vi "Start.vi"(8 "error in (no error)":errorcluster, 10 "Message in":refnum<class "StartMessage.lvclass">, 11 "Waveform in":refnum<class "Waveform.lvclass">) -> (0 "error out":errorcluster, 3 "Waveform out":refnum<class "Waveform.lvclass">)   [LabVIEW 2012, in "Waveform.lvclass"]
doc: "This member function is called when the statemachine in the run.vi receives an 'start' command. It relays the message to all observers of the component.\n\nOverride this member function in your derived class if you need additional start functionality (but don't forget to call the parent method)."
uses:
  Waveform.lvclass
  <vilib>/Distrio/Murmex/StartMessage/StartMessage.lvclass
  <vilib>/Distrio/Murmex/Murmex/Murmex.lvclass
  <vilib>/Distrio/Murmex/StartMessage/run mode enum.ctl
  Waveform.lvclass/Waveform.ctl
  <vilib>/Distrio/Murmex/StartMessage/Get run mode.vi
  <vilib>/Distrio/Murmex/Message/Message.lvclass
panel:
  # "This member function is called when the statemachine in the run.vi receives an 'start' command. It relays the message to all observers of the component.\n\nOverride this member function in your derived class if you need additional start functionality (but don't forget to call the parent method)."
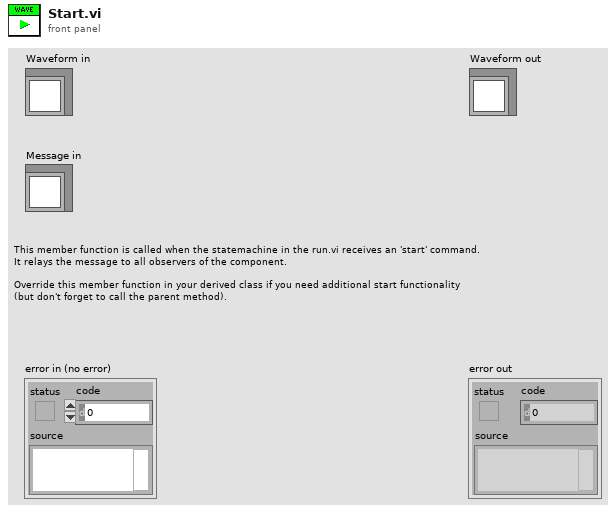
[diagram p1: front panel]
types:
  T1 = enum8{"Enabled", "Disabled", "Disabled and Grayed Out"}
  T2 = typedef "Murmex.lvlib/StartMessage.lvclass/run mode enum.ctl" = enum16{"infinite", "finite"}
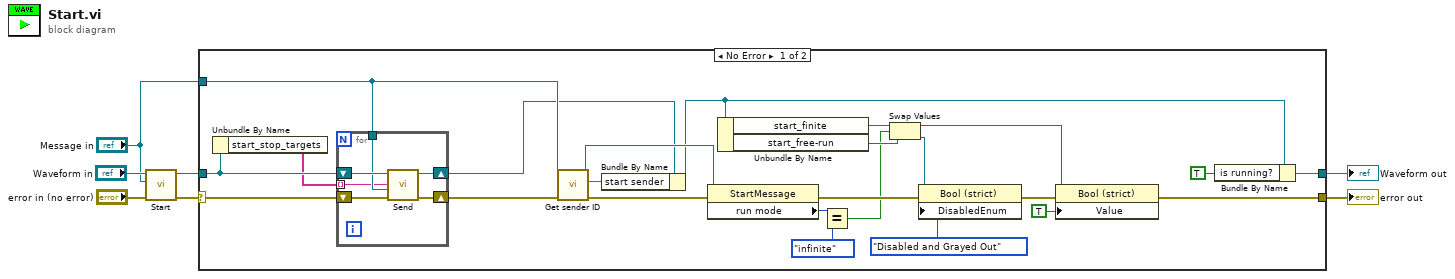
[diagram p0: block diagram]
diagram:
  n1 = call-parent "Start.vi"("error in (no error)"="error in (no error)", "Message in"="Message in", "Murmex in"="Waveform in") -> ("error out"=w5:errorcluster, "Murmex out"=w4:refnum<class "Waveform.lvclass">)  [unwired: 7 in]
  n2 = case shown="No Error" w5 {
    selector: w5 -> [w16 w39]
    tunnel: w4 -> [w14 w38]
    tunnel: [w9 w39] -> w3
    tunnel: [w17 w38] -> w2
    tunnel: "Message in" -> [w15 _]
    frame No Error {
      n3 = Unbundle By Name(w14) -> ("start_stop_targets"=w13:string[])
      n4 = for {
        shift-right: [w36] -> w11
        shift-left: w16 -> [w37]
        shift-right: [w34] -> w10
        shift-left: w14 -> [w35]
        tunnel: w15 -> [w33]
        tunnel: w13 -> [w32] mode=indexing
        n5 = call <vilib>:"Send.vi"("error in (no error)"=w37, "Message"=w33, "recipient"=w32, "Murmex in"=w35) -> ("error out"=w36:errorcluster, "Murmex out"=w34:refnum<class "Waveform.lvclass">)  [unwired: 6 in]
      }
      n6 = call <vilib>:"Get sender ID.vi"("error in (no error)"=w11, "Message in"=w15) -> ("error out"=w30:errorcluster, "sender"=w31:string, "Message out"=w29:refnum<class "StartMessage.lvclass">)  [unwired: 7 in]
      n7 = Bundle By Name(cluster=w10, "start sender"=w31) -> (w8:refnum<class "Waveform.lvclass">)
      n8 = property class="StartMessage"(reference=w29, error in=w30) -> (error out=w23:errorcluster, "run mode"=w19:T2)  [unwired: 1 out]
      n9 = Unbundle By Name(w8) -> ("start_finite"=w27:refnum<vi>, "start_free-run"=w26:refnum<vi>)
      n10 = Equal?(x=w19, y=run_mode_enum."infinite" ("run mode")) -> (x = y?=w12:bool)
      n11 = Swap Values(12:w27, 13:w12, 14:w26) -> (1:w24:refnum<vi>, 3:w25:refnum<vi>)
      n12 = property class="Bool (strict)"(reference=w25, error in=w23, "DisabledEnum"=T1."Disabled and Grayed Out" ("Disabled")) -> (error out=w22:errorcluster)  [unwired: 1 out]
      n13 = property class="Bool (strict)"(reference=w24, error in=w22, "Value"=TRUE) -> (error out=w9:errorcluster)  [unwired: 1 out]
      n14 = Bundle By Name(cluster=w8, "is running?"=TRUE ("runtime.is running?")) -> (w17:refnum<class "Waveform.lvclass">)
    }
    frame Error {
    }
  }
  "error out" <- w3
  "Waveform out" <- w2
